vi "save_decrement.vi"(8 "error in (no error)":errorcluster, 11 "HGF_Reference":refnum<class "HGF_Reference.lvclass">) -> (0 "error out":errorcluster, 3 "dup HGF_Reference":refnum<class "HGF_Reference.lvclass">)   [LabVIEW 2009, in "HB_BaseClass_Examples.lvlib" / "HB_Simple.lvclass"]
doc: "This VI provides a method to decrement the referenced object attribute with giving direct access to it wire."
uses:
  HB_Simple.lvclass
  lib.lib/HGF_LVC/HGF_BaseClasses/HGF_Reference/HGF_Reference.lvclass
panel:
  in  "timeout in ms (-1)":i32=-1
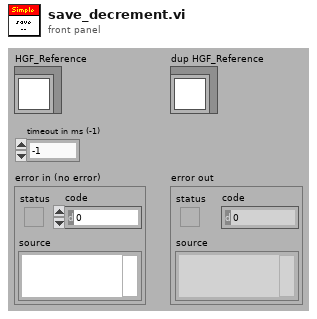
[diagram p1: front panel]
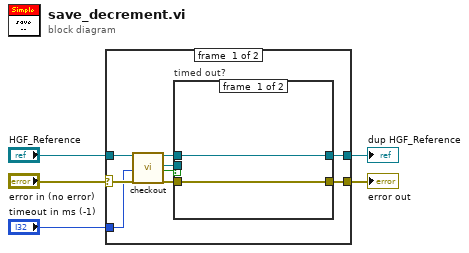
[diagram p0: block diagram]
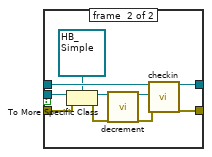
[diagram p2: hidden frame]
diagram:
  n1 = case shown="No Error" "error in (no error)" {
    selector: "error in (no error)" -> [w8 w28]
    tunnel: [w7 w28] -> w4
    tunnel: [w10 w27] -> w2
    tunnel: "HGF_Reference" -> [w11 w27]
    tunnel: "timeout in ms (-1)" -> [w6 _]
    frame #0 {
      n2 = call "checkout.vi"("HGF_Reference"=w11, "timeout in ms (-1)"=w6, "error in (no error)"=w8) -> ("dup HGF_Reference"=w14:refnum<class "HGF_Reference.lvclass">, "Object"=w12:refnum<class>, "got object?"=w9:bool, "error out"=w13:errorcluster)  [unwired: 13 out]
      n3 = case "timed out?" shown="True" w9 {
        tunnel: w14 -> [w16 w26]
        tunnel: w13 -> [w15 w25]
        tunnel: w12 -> [_ w24]
        tunnel: [w16 w18] -> w10
        tunnel: [w15 w17] -> w7
        frame #0 {
        }
        frame #1 {
          n4 = To More Specific Class(target class=refnum<class "HB_Simple.lvclass"> refnum ("HB_Simple in"), reference=w24, error in=w25) -> (specific class reference=w23:refnum<class "HB_Simple.lvclass">, error out=w21:errorcluster)
          n5 = call "decrement.vi"("HB_Simple in"=w23, "error in (no error)"=w21) -> ("HB_Simple out"=w22:refnum<class "HB_Simple.lvclass">, "error out"=w20:errorcluster)  [unwired: 16 in]
          n6 = call "checkin.vi"("HGF_Reference"=w26, "Object"=w22, "error in (no error)"=w20) -> ("dup HGF_Reference"=w18:refnum<class "HGF_Reference.lvclass">, "error out"=w17:errorcluster)  [unwired: 1 in, 14 out]
        }
      }
    }
    frame #1 {
    }
  }
  "error out" <- w4
  "dup HGF_Reference" <- w2
